vi "Concatenate Signal Records.vi"(4 "Signal Record Array":waveform(dbl)[][](array[waveform])) -> (1 "Concatenated Signals":waveform(dbl)[](array[waveform]))   [LabVIEW 2013]
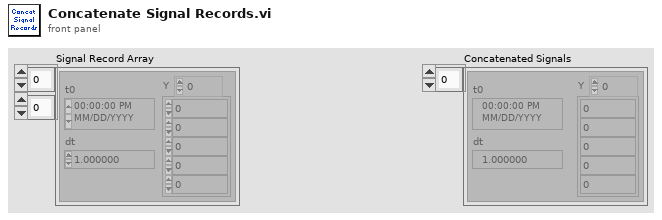
[diagram p1: front panel]
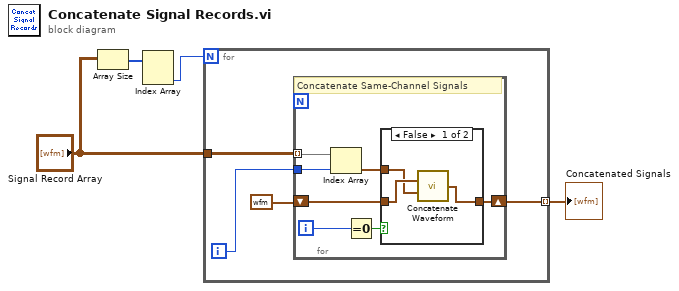
[diagram p0: block diagram]
diagram:
  n1 = Array Size(array="Signal Record Array") -> (size(s)=w4:i32[])
  n2 = Index Array(array=w4) -> (element #2=w3:i32)  [unwired: 2 in, 1 out]
  n3 = for {
    N: w3 -> [_]
    tunnel: "Signal Record Array" -> [w8]
    tunnel: [w5] -> w1 mode=indexing
    i -> [w7]
    n4 = for {
      tunnel: w8 -> [w13] mode=indexing
      shift-right: [w10] -> w5
      shift-left: waveform(dbl) {"t0"=timestamp(0 s since 1904-01-01), "dt"=1.0, "Y"=[]} ("Waveform") -> [w9]
      tunnel: w7 -> [w12]
      i -> [w14]
      # "Concatenate Same-Channel Signals"
      n5 = Index Array(array=w13, index=w12) -> (element=w11:waveform(dbl))
      n6 = Equal To 0?(x=w14) -> (x = 0?=w15:bool)
      n7 = case shown="False" w15 {
        tunnel: w11 -> [w16 w19]
        tunnel: [w18 w19] -> w10
        tunnel: w9 -> [w17 _]
        frame False {
          n8 = call "Concatenate Waveform.vi"("Base Waveform"=w17, "Waveform"=w16) -> ("Concatenated Waveform"=w18:waveform(dbl))  [unwired: 13 in]
        }
        frame True {
        }
      }
    }
  }
  "Concatenated Signals" <- w1
